vi "x-y plot current point and history clustors.vi"(6 "clear?":bool, 10 "Y":dbl[](array[numeric]), 11 "X":dbl[](array[numeric])) -> (2 "History":cluster{dbl[], dbl[]}, 3 "Current Point":cluster{"Zi":dbl[], "Zi":dbl[]})   [LabVIEW 2020]
doc: "Creates clustors containing the current x-y point and the x-y point history. Preallocated clone execution means that each instance of this subVI keeps it's own history in un-initialized shift registers."
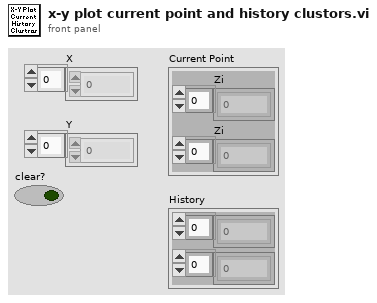
[diagram p1: front panel]
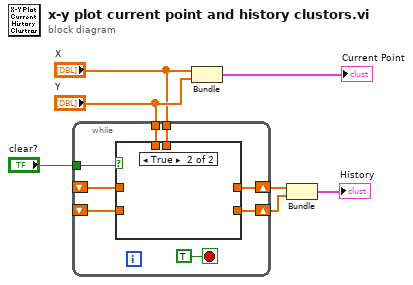
[diagram p0: block diagram]
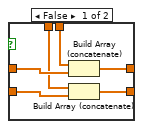
[diagram p2: hidden frame]
diagram:
  n1 = while {
    shift-right: [w14] -> w2
    shift-left: _ -> [w13]
    shift-right: [w12] -> w3
    shift-left: _ -> [w11]
    tunnel: "X" -> [w10]
    tunnel: "Y" -> [w9]
    tunnel: "clear?" -> [w8]
    stop <- TRUE stop-if-true
    n2 = case shown="True" w8 {
      tunnel: [w21 _] -> w14
      tunnel: w13 -> [w20 _]
      tunnel: [w19 _] -> w12
      tunnel: w11 -> [w18 _]
      tunnel: w10 -> [w17 _]
      tunnel: w9 -> [w16 _]
      frame False {
        n3 = Build Array (concatenate)(w17, w20) -> (w21:dbl[])
        n4 = Build Array (concatenate)(w16, w18) -> (w19:dbl[])
      }
      frame True {
      }
    }
  }
  n5 = Bundle("X"="X", "Y"="Y") -> (→"Current Point":cluster{"X":dbl[], "Y":dbl[]})  [unwired: 1 in]
  n6 = Bundle(w2, w3) -> (→"History":cluster{dbl[], dbl[]})  [unwired: 1 in]
